vi "Plot subChangeDetector.vi"(10 "value":variant) -> (1 "changed?":bool, 2 "previous value":variant)   [LabVIEW 2020, in "2D Plot.lvclass"]
uses:
  <vilib>/Math Plots/2D Math Plots/2D Plot/2D Plot/2D Plot.lvclass
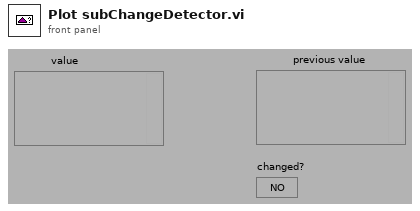
[diagram p1: front panel]
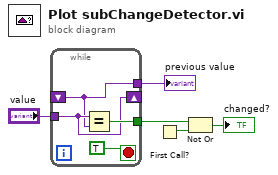
[diagram p0: block diagram]
diagram:
  n1 = while {
    tunnel: [w8] -> w5
    shift-left: _ -> [w6]
    shift-right: [w7] -> _
    tunnel: "value" -> [w7]
    tunnel: [w6] -> w1
    stop <- TRUE stop-if-true
    n2 = Equal?(x=w7, y=w6) -> (x = y?=w8:bool)
  }
  "previous value" <- w1
  n3 = First Call?() -> (First Call?: T/F=w4:bool)
  n4 = Not Or(1:w4, 2:w5) -> (0:→"changed?":bool)
